vi "ma_SML Spectrum Unit Conversion.vi"(4 "window":u16(ring) items=["Rectangle"=0, "Hanning"=1, "Hamming"=2, "Blackman-Harris"=3, "Exact Blackman"=4, "Blackman"=5, "Flat Top"=6, "4 Term B-Harris "=7, "7 Term B-Harris"=8, "Low Sidelobe"=9, "Blackman Nuttall"=11, "Triangle"=30, "Bartlett-Hanning"=31, "Bohman"=32, "Parzen"=33, "Welch"=34, "Kaiser"=60, "Dolph-Chebyshev"=61, "Gaussian"=62], 5 "dB and ref.":T1={"log/linear"=enum."Linear", "reference unit"=enum."uV", "impedance(ohm)"=600.0, "scaling"=enum."rms"} {"impedance(ohm)" format="%.2f"}, 6 "zero padding ratio":dbl=1.0 format="%.2f", 7 "spectrum type":T2(ring), 8 "df":dbl=1.0 format="%.2f", 9 "spectrum":dbl[](array[numeric]) format="%.2f") -> (0 "spectrum unit":string="dBVpk", 3 "spectrum":dbl[](array[numeric]) format="%.5f")   [LabVIEW 2020, in "NI_MAPro.lvlib"]
doc: "Converts the input spectrum (power, amplitude, or gain) to alternate formats including Log (dB or dBm) and spectral density.\n\nSpectrum is the input array containing a spectrum of the type specified by the spectrum type selector:\n spectrum type = 0 Power (Vrms^2)\n spectrum type = 1 Amplitude (Vrms)\n spectrum type = 2 Gain (amplitude ratio)\n\nThe signal unit (V) string control specifies the units of the spectrum. The signal unit (V) control defaults to V (volts).\n\nThe log/linear control has three selections for the output unit type\n log/linear = 0 Linear\n log/linear = 1 dB\n log/linear = 2 dBm\n\nThe display unit has the following selections for the display unit:\n 0: Vrms (volts rms)\n 1: Vpk (volts peak)\n 2: Vrms^2 (volts squared rms)\n 3: Vpk^2 (volts squared peak)\n 4: Vrms/ÃHz (volts rms per root Hz)\n 5: Vpk/ÃHz (volts peak per root Hz)\n 6: Vrms^2/Hz (volts squared rms per Hz)\n 7: Vpk^2/Hz (volts squared peak per Hz)\n\nThe last four selections are amplitude spectral density (4,5) and power spectral density (6,7).\nThe control cluster window constants contains constants for the selected window (from the Scaled Time Domain Window VI). You need this input only when you use the spectral density output formats (the last four output unit selections)."
uses:
  NI_MAPro.lvlib
panel:
  # "SML Spectrum Unit Conversion"
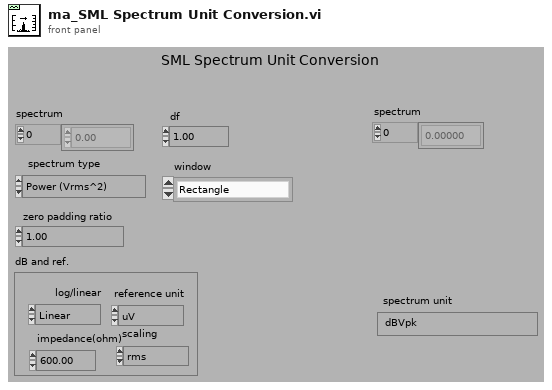
[diagram p1: front panel]
types:
  T1 = cluster{"log/linear":enum16{"Linear", "dB"}, "reference unit":enum16{"V", "mV", "uV", "W", "mW", "uW"}, "impedance(ohm)":dbl, "scaling":enum16{"rms", "pk", "rms^2", "pk^2", "rms/rtHz", "pk/rtHz", "rms^2/Hz", "pk^2/Hz"}}
  T2 = enum16{"Power (Vrms^2)", "Amplitude (Vrms)", "Gain (amplitude ratio)"}
  T3 = enum16{"rms", "pk", "rms^2", "pk^2", "rms/rtHz", "pk/rtHz", "rms^2/Hz", "pk^2/Hz"}
  T4 = enum32{"rms", "pk", "rms^2", "pk^2", "rms/rtHz", "pk/rtHz", "rms^2/Hz", "pk^2/Hz"}
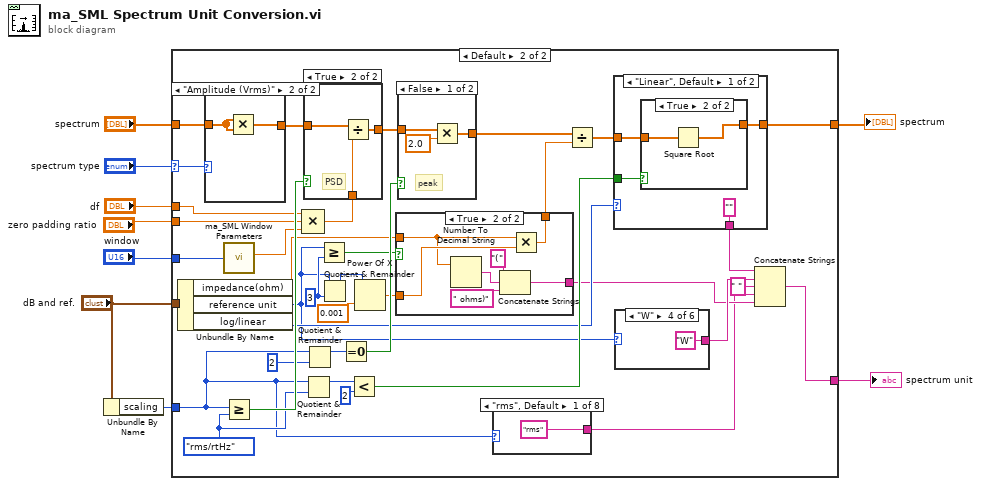
[diagram p0: block diagram]
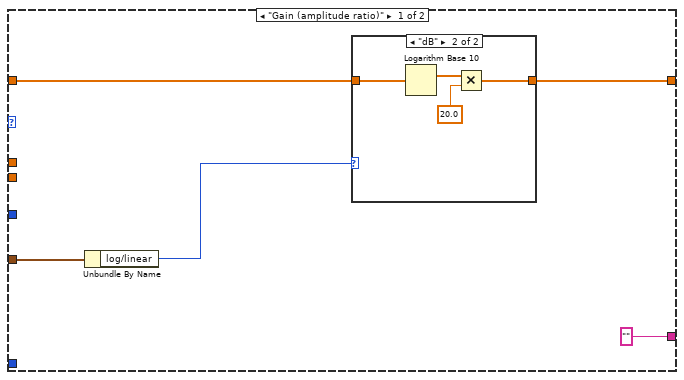
[diagram p2: hidden frame]
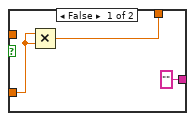
[diagram p4: hidden frame]
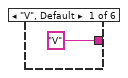
[diagram p5: hidden frame]
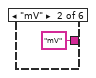
[diagram p6: hidden frame]
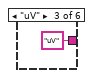
[diagram p7: hidden frame]
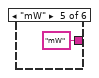
[diagram p8: hidden frame]
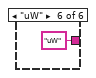
[diagram p9: hidden frame]
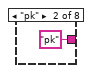
[diagram p10: hidden frame]
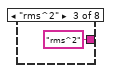
[diagram p11: hidden frame]
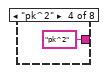
[diagram p12: hidden frame]
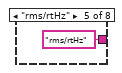
[diagram p13: hidden frame]
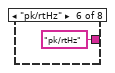
[diagram p14: hidden frame]
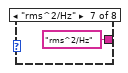
[diagram p15: hidden frame]
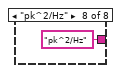
[diagram p16: hidden frame]
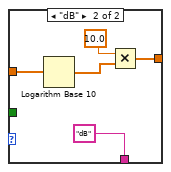
[diagram p18: hidden frame]
diagram:
  n1 = Unbundle By Name("dB and ref.") -> ("scaling"=w2:T3)
  n2 = case shown="Default" "spectrum type" {
    selector: "spectrum type" -> [_ w56]
    tunnel: "dB and ref." -> [w14 w42]
    tunnel: "spectrum" -> [w12 w55]
    tunnel: [w11 w36] -> w6
    tunnel: ["" ("spectrum unit") w26] -> w5
    tunnel: w2 -> [_ w23]
    tunnel: "df" -> [_ w52]
    tunnel: "window" -> [_ w20]
    tunnel: "zero padding ratio" -> [_ w22]
    frame "Gain (amplitude ratio)" {
      n3 = Unbundle By Name(w14) -> ("log/linear"=w13:enum16{"Linear", "dB"})
      n4 = case shown="\"dB\"" w13 {
        tunnel: w12 -> [w15 w19]
        tunnel: [w15 w18] -> w11
        frame "Linear", Default {
        }
        frame "dB" {
          n5 = Logarithm Base 10(1:w19) -> (0:w17:dbl[])
          n6 = Multiply(x=w17, y=20.0) -> (x*y=w18:dbl[])
        }
      }
    }
    frame Default {
      w39 = u32 3 ("y")
      w50 = T4."rms/rtHz" ("y")
      n7 = Unbundle By Name(w42) -> ("impedance(ohm)"=w31:dbl, "reference unit"=w33:enum16{"V", "mV", "uV", "W", "mW", "uW"}, "log/linear"=w34:enum16{"Linear", "dB"})
      n8 = case shown="\"Amplitude (Vrms)\"" w56 {
        tunnel: w55 -> [w101 w103]
        tunnel: [w101 w102] -> w53
        frame "Power (Vrms^2)", Default {
        }
        frame "Amplitude (Vrms)" {
          n9 = Multiply(x=w103, y=w103) -> (x*y=w102:dbl[])
        }
      }
      n10 = call "ma_SML Window Parameters.vi"("window"=w20) -> ("ENBW"=w21:dbl)  [unwired: 3 out]
      n11 = Greater Or Equal?(x=w23, y=w50) -> (x >= y?=w54:bool)
      n12 = Compound Arithmetic op=MULTIPLY(w52, w22, w21) -> (w51:dbl)
      n13 = case shown="True" w54 {
        tunnel: w53 -> [w97 w100]
        tunnel: w51 -> [_ w99]
        tunnel: [w97 w98] -> w44
        frame False {
          # "power"
        }
        frame True {
          # "PSD"
          n14 = Divide(x=w100, y=w99) -> (x/y=w98:dbl[])
        }
      }
      n15 = Quotient & Remainder(x=w23, y=w50) -> (x-y*floor(x/y)=w49:u32)  [unwired: 1 out]
      n16 = Quotient & Remainder(x=w23, y=2) -> (x-y*floor(x/y)=w46:i32)  [unwired: 1 out]
      n17 = Greater Or Equal?(x=w33, y=w39) -> (x >= y?=w32:bool)
      n18 = Quotient & Remainder(x=w33, y=w39) -> (x-y*floor(x/y)=w41:u32)  [unwired: 1 out]
      n19 = Equal To 0?(x=w46) -> (x = 0?=w45:bool)
      n20 = Less?(x=w49, y=u32 2) -> (x < y?=w38:bool)
      n21 = Power Of X(1:0.001 ("x"), 2:w41) -> (0:w35:dbl)
      n22 = case shown="True" w32 {
        tunnel: w35 -> [w59 w66]
        tunnel: w31 -> [_ w61]
        tunnel: [w58 w65] -> w30
        tunnel: ["" w60] -> w27
        frame False {
          n23 = Multiply(x=w59, y=w59) -> (x*y=w58:dbl)
        }
        frame True {
          n24 = Number To Decimal String(number=w61) -> (decimal integer string=w62:string)  [unwired: 1 out]
          n25 = Concatenate Strings("(" ("Substring"), w62, " ohms)" ("Substring")) -> (w60:string)
          n26 = Multiply(x=w61, y=w66) -> (x*y=w65:dbl)
        }
      }
      n27 = case shown="False" w45 {
        tunnel: w44 -> [w94 w96]
        tunnel: [w93 w96] -> w43
        frame False {
          # "peak"
          n28 = Multiply(x=w94, y=2.0) -> (x*y=w93:dbl[])
        }
        frame True {
        }
      }
      n29 = case shown="\"rms\", Default" w23 {
        tunnel: ["rms" ("spectrum unit") "pk" ("spectrum unit") "rms^2" ("spectrum unit") "pk^2" ("spectrum unit") "rms/rtHz" ("spectrum unit") "pk/rtHz" ("spectrum unit") "rms^2/Hz" ("spectrum unit") "pk^2/Hz" ("spectrum unit")] -> w25
        frame "rms", Default {
        }
        frame "pk" {
        }
        frame "rms^2" {
        }
        frame "pk^2" {
        }
        frame "rms/rtHz" {
        }
        frame "pk/rtHz" {
        }
        frame "rms^2/Hz" {
        }
        frame "pk^2/Hz" {
        }
      }
      n30 = Divide(x=w43, y=w30) -> (x/y=w37:dbl[])
      n31 = case shown="\"Linear\", Default" w34 {
        tunnel: w38 -> [w84 _]
        tunnel: w37 -> [w83 w92]
        tunnel: [w82 w91] -> w36
        tunnel: ["" "dB"] -> w29
        frame "Linear", Default {
          n32 = case shown="True" w84 {
            tunnel: w83 -> [w85 w87]
            tunnel: [w85 w86] -> w82
            frame False {
            }
            frame True {
              n33 = Square Root(x=w87) -> (sqrt(x)=w86:dbl[])
            }
          }
        }
        frame "dB" {
          n34 = Logarithm Base 10(1:w92) -> (0:w90:dbl[])
          n35 = Multiply(x=10.0, y=w90) -> (x*y=w91:dbl[])
        }
      }
      n36 = case shown="\"W\"" w33 {
        tunnel: ["V" ("spectrum unit") "mV" ("spectrum unit") "uV" ("spectrum unit") "W" ("spectrum unit") "mW" ("spectrum unit") "uW" ("spectrum unit")] -> w28
        frame "V", Default {
        }
        frame "mV" {
        }
        frame "uV" {
        }
        frame "W" {
        }
        frame "mW" {
        }
        frame "uW" {
        }
      }
      n37 = Concatenate Strings(w29, w28, " " ("Substring"), w25, w27) -> (w26:string)
    }
  }
  "spectrum unit" <- w5
  "spectrum" <- w6
